vi "StartEditor.vi"(11 "CodeEditorRef":refnum<k24>) -> ()   [LabVIEW 2020]
uses:
  C:/Users/User/Desktop/Automation/CurrentVersion/LabviewDXFViewer/bin/Release/LabviewDXFViewer.exe
  LabviewDXFViewer/bin/Release/LabviewDXFViewer.exe
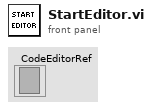
[diagram p1: front panel]
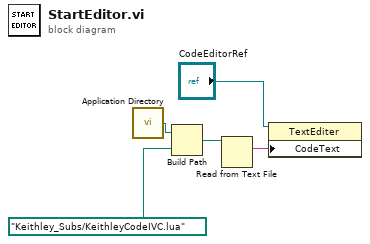
[diagram p0: block diagram]
diagram:
  n1 = call <vilib>:"Application Directory.vi"() -> ("Application Directory"=w3:path)
  n2 = Build Path(base path=w3, name or relative path=path "Keithley_Subs/KeithleyCodeIVC.lua" ("file (use dialog)")) -> (appended path=w5:path)
  n3 = Read from Text File(file (use dialog)=w5) -> (text=w2:string)  [unwired: 3 in, 3 out]
  n4 = property class="TextEditer"(reference="CodeEditorRef", "CodeText"=w2) -> ()  [unwired: 1 in, 2 out]
